vi "ifr2025 Select.vi"(8 "error in (no error)":errorcluster {"code" format="%.0x"}, 9 "Select (OFF)":i16(ring) items=["OFF", "SEQ1", "SEQ2", "SEQ3", "SEQ4", "SEQ5", "SEQ6", "SEQ7", "SEQ8", "SEQ9"], 11 "instrument handle":refnum<visa-resource-name>) -> (0 "error out":errorcluster {"code" format="%.0x"}, 1 "Stop":i16, 2 "Start":i16, 3 "instrument handle out":refnum<visa-resource-name>)   [LabVIEW 2009]
doc: "This command allows one of the nine sequences to be defined as the current sequence."
uses:
  Ifr2025_32.dll
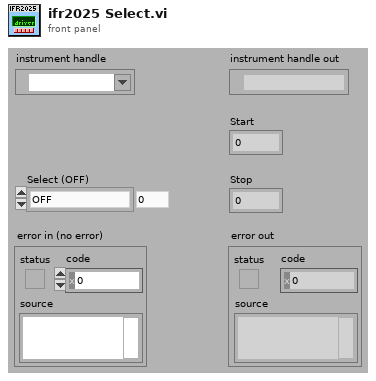
[diagram p1: front panel]
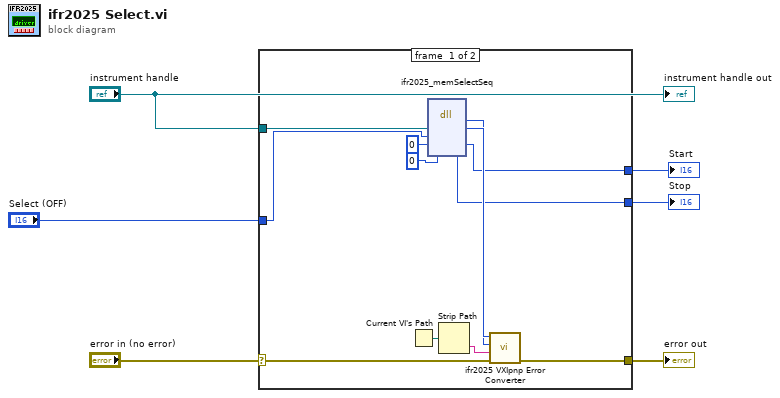
[diagram p0: block diagram]
diagram:
  n1 = case shown="No Error" "error in (no error)" {
    selector: "error in (no error)" -> [w13 w19]
    tunnel: [w12 w19] -> w6
    tunnel: "instrument handle" -> [w17 _]
    tunnel: "Select (OFF)" -> [w11 _]
    tunnel: [w9 _] -> w2
    tunnel: [w7 _] -> w1
    frame #0 {
      n2 = Current VI's Path() -> (path=w18:path)
      n3 = dll-call lib="P:/inst/Marconi 2024 Signal Generator/source/labview/ifr2025/ifr2025/ifr2025_*.*" fn="ifr2025_memSelectSeq"("vi"=w17, "Select"=w11, "Start"=i16 0, "Stop"=i16 0) -> (w15:i32, "vi"=w16:u32, "Start"=w9:i16, "Stop"=w7:i16)  [unwired: 4 in, 2 out]
      n4 = Strip Path(path=w18) -> (name=w14:string)  [unwired: 1 out]
      n5 = call "ifr2025 VXIpnp Error Converter.vi"("error in (no error)"=w13, "name of VI (\"\")"=w14, "CVI error code (0)"=w15, "instrument handle"=w16) -> ("error out"=w12:errorcluster)  [unwired: 7 out]
    }
    frame #1 {
    }
  }
  "error out" <- w6
  "Start" <- w2
  "Stop" <- w1
  "instrument handle out" <- "instrument handle"
